vi "niRFUtil LCAPI Copy WFM (2 SGL).vi"(0 "Source0 WFM (SGL)":T1 {"y" min=0 max=127 format="%.2f"; "dx" format="%^.2e"; "x0" format="%^.2e"}, 5 "Source1 WFM (SGL)":T1 {"y" min=0 max=127 format="%.2f"; "dx" format="%^.2e"; "x0" format="%^.2e"}, 11 "error in (no error)":errorcluster, 12 "Data Copy Descriptor":u64) -> (4 "Source0 Out":T1 {"y" min=0 max=127 format="%.2f"; "dx" format="%^.2e"; "x0" format="%^.2e"}, 6 "Source1 Out":T1 {"y" min=0 max=127 format="%.2f"; "dx" format="%^.2e"; "x0" format="%^.2e"}, 15 "error out":errorcluster)   [LabVIEW 2015, in "niRFUtil.lvlib"]
uses:
  niRFUtil.lvlib
  Includes/niRFUtil INC Real Waveform.ctl
  Includes/niRFUtil INC Real Array.ctl
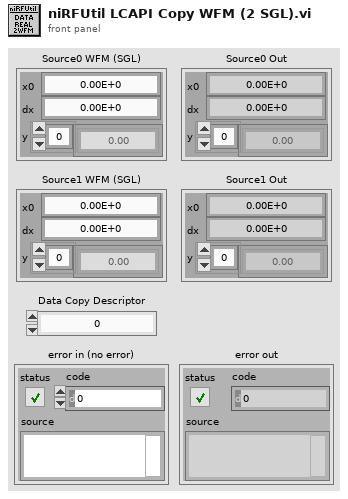
[diagram p1: front panel]
types:
  T1 = typedef "niRFUtil.lvlib/niRFUtil INC Real Waveform.ctl" = cluster{"x0":dbl, "dx":dbl, "y":T2}
  T2 = typedef "niRFUtil.lvlib/niRFUtil INC Real Array.ctl" = sgl[]
  T3 = cluster{"status":bool, "return type":i32, "errorString":string}
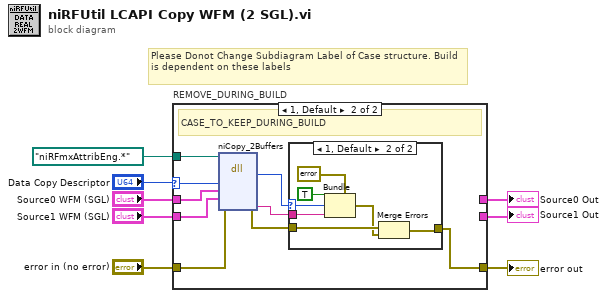
[diagram p0: block diagram]
diagram:
  # "Please Donot Change Subdiagram Label of Case structure. Build is dependent on these labels"
  n1 = case "REMOVE_DURING_BUILD" shown="1, Default" "Data Copy Descriptor" {
    selector: "Data Copy Descriptor" -> [_ w14]
    tunnel: "Source0 WFM (SGL)" -> [w11 w20]
    tunnel: "error in (no error)" -> [w9 w19]
    tunnel: "Source1 WFM (SGL)" -> [w10 w18]
    tunnel: [w11 _] -> w4
    tunnel: [w10 _] -> w3
    tunnel: [w9 w13] -> w2
    tunnel: path "niRFmxAttribEng.*" ("path in") -> [_ w12]
    frame 0 {
      # "Development"
    }
    frame 1, Default {
      # "CASE_TO_KEEP_DURING_BUILD"
      n2 = dll-call lib="niRFmxAttribEng.*" fn="niCopy_2Buffers"(path in=w12, error in=w19, "dataCopyDescriptor"=w14, "source0"=w20, "source1"=w18) -> (error out=w15:errorcluster, "return type"=w16:i32, "errorString"=w17:string)  [unwired: 5 in, 1 out]
      n3 = case shown="1, Default" w16 {
        selector: w16 -> [_ w25]
        tunnel: w17 -> [_ w26]
        tunnel: w15 -> [w21 w28]
        tunnel: [w21 w27] -> w13
        frame 0 {
        }
        frame 1, Default {
          n4 = Bundle(cluster=T3 {"status"=FALSE, "return type"=0, "errorString"=""}, "status"=TRUE, "return type"=w25, "errorString"=w26) -> (w22:T3)
          n5 = Merge Errors(w28, w22) -> (w27:errorcluster)
        }
      }
    }
  }
  "error out" <- w2
  "Source0 Out" <- w4
  "Source1 Out" <- w3
